vi "Match motor to input.vi"(9 "start time":timestamp, 10 "motor":waveform(dbl), 11 "voltage":waveform(dbl)[](array[waveform])) -> (2 "time":dbl, 3 "motor subset":waveform(dbl))   [LabVIEW 2013]
uses:
  <vilib>/Waveform/WDTOps.llb/WDT Waveform Duration DBL.vi
  <vilib>/Waveform/WDTOps.llb/WDT Get Waveform Subset DBL.vi
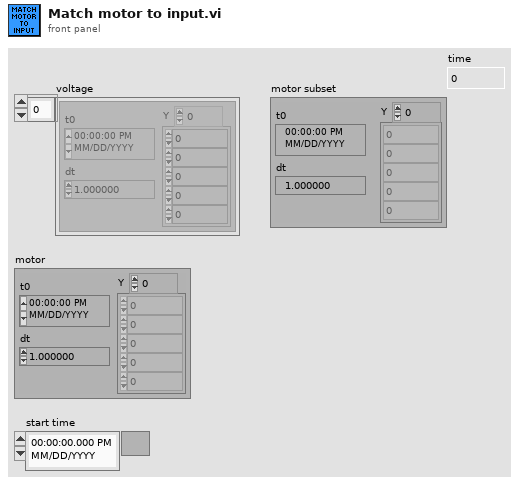
[diagram p1: front panel]
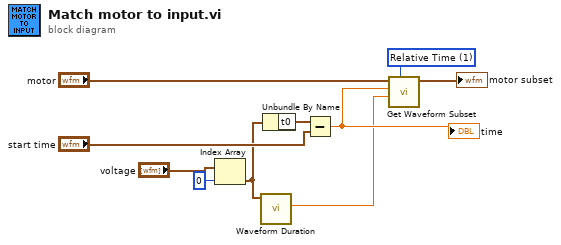
[diagram p0: block diagram]
diagram:
  w4 = u16 1 items=["Samples", "Relative Time"] ("start/duration format")
  n1 = Index Array(array="voltage", index=0) -> (element=w2:waveform(dbl))
  n2 = call-poly <vilib>:"Waveform Duration.vi"("waveform in"=w2) -> ("duration"=w5:dbl)  [unwired: 8 in, 2 out]
  n3 = Unbundle By Name(w2) -> ("t0"=w6:timestamp)
  n4 = Subtract(x=w6, y="start time") -> (x-y=w8:dbl)
  "time" <- w8
  n5 = call-poly <vilib>:"Get Waveform Subset.vi"("start/duration format"=w4, "duration"=w5, "start samples/time"=w8, "waveform in"="motor") -> ("waveform out"=→"motor subset":waveform(dbl))  [unwired: 2 in, 3 out]
